vi "Data Parsing.vi"(8 "error in":errorcluster, 10 "Data Read":string, 11 "Modbus in":refnum<class "Modbus.lvclass">) -> (0 "error out":errorcluster, 1 "Graph Data":T1, 2 "Data Out":string[](array[string]), 3 "Modbus out":refnum<class "Modbus.lvclass">)   [LabVIEW 2021, in "Modbus.lvclass"]
uses:
  Modbus.lvclass
  controls/Data for Graph.ctl
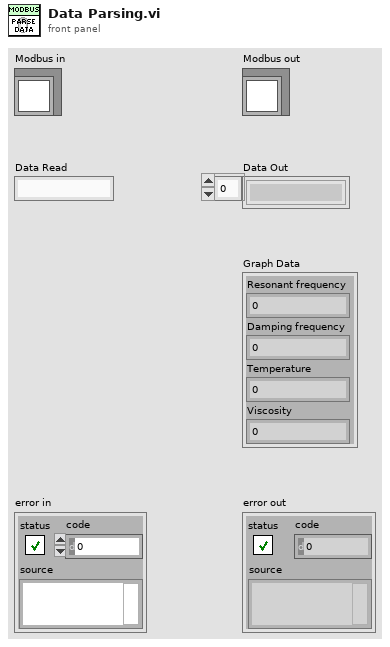
[diagram p1: front panel]
types:
  T1 = typedef "Data for Graph.ctl" = cluster{"Resonant frequency":dbl, "Damping frequency":dbl, "Temperature":dbl, "Viscosity":dbl}
  T2 = enum16{"big-endian, network order", "native, host order", "little-endian"}
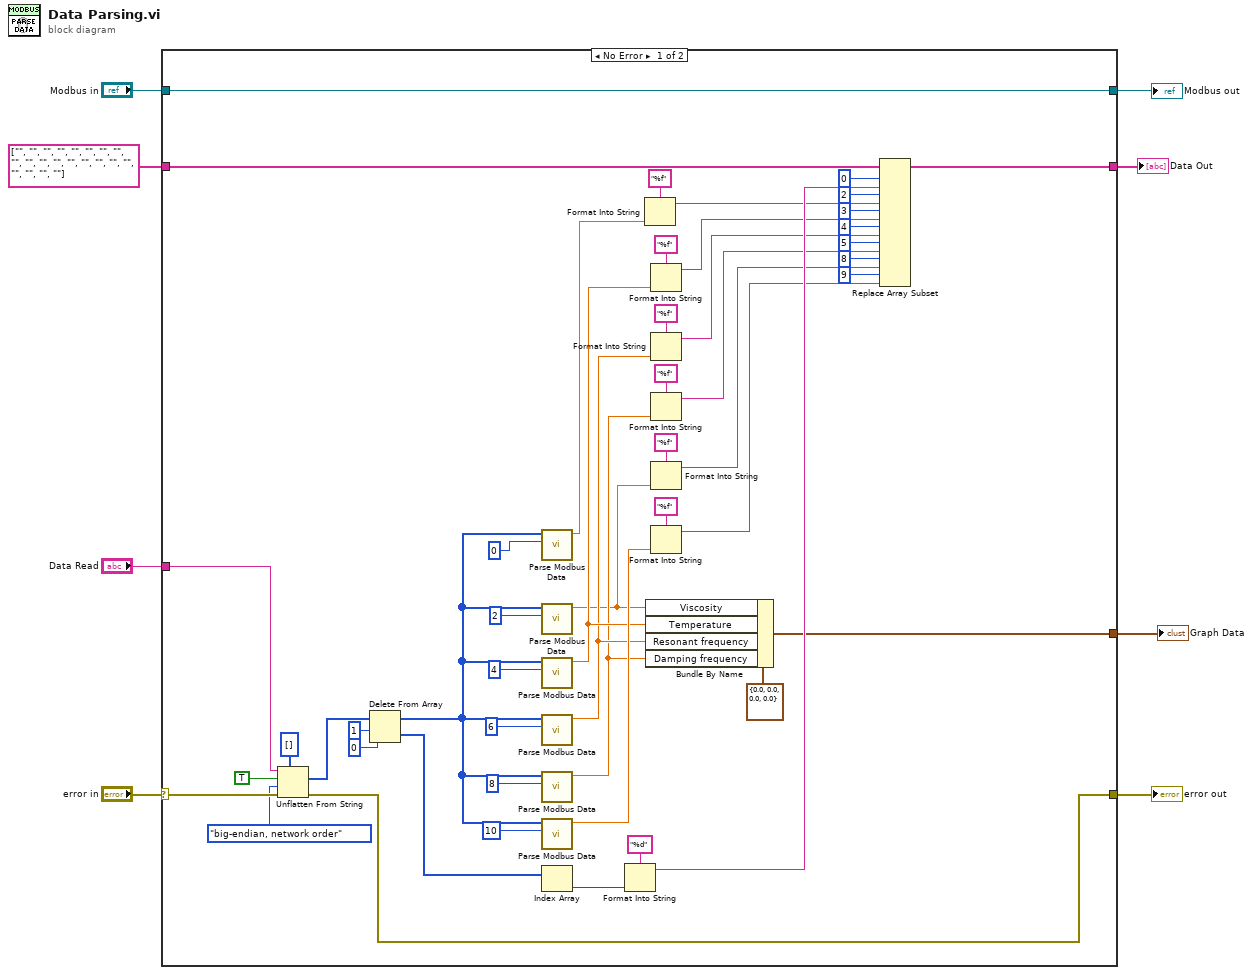
[diagram p0: block diagram]
diagram:
  n1 = case shown="No Error" "error in" {
    selector: "error in" -> [w53 w59]
    tunnel: [w38 w59] -> w7
    tunnel: "Modbus in" -> [w56 w60]
    tunnel: [w56 w60] -> w5
    tunnel: "Data Read" -> [w55 _]
    tunnel: [w39 _] -> w3
    tunnel: string[] ["", "", "", "", "", "", "", "", "", "", "", "", "", "", "", "", "", "", "", "", ""] -> [w37 _]
    tunnel: [w16 _] -> w1
    frame No Error {
      n2 = Unflatten From String(type=u16[] [] ("register values"), binary string=w55, data includes array or string size? (T)=TRUE, byte order (0:big-endian, network order)=T2."big-endian, network order", error in (no error)=w53) -> (value=w50:u16[], error out=w38:errorcluster)  [unwired: 1 out]
      n3 = Delete From Array(array=w50, length=1, index=0) -> (deleted portion=w36:u16[], array with subset deleted=w42:u16[])
      n4 = call "Parse Modbus Data.vi"("Start Index"=0, "Register Data"=w42) -> ("Result"=w32:dbl)  [unwired: 9 in]
      n5 = call "Parse Modbus Data.vi"("Start Index"=2, "Register Data"=w42) -> ("Result"=w19:dbl)  [unwired: 9 in]
      n6 = call "Parse Modbus Data.vi"("Start Index"=4, "Register Data"=w42) -> ("Result"=w25:dbl)  [unwired: 9 in]
      n7 = call "Parse Modbus Data.vi"("Start Index"=6, "Register Data"=w42) -> ("Result"=w24:dbl)  [unwired: 9 in]
      n8 = call "Parse Modbus Data.vi"("Start Index"=8, "Register Data"=w42) -> ("Result"=w23:dbl)  [unwired: 9 in]
      n9 = call "Parse Modbus Data.vi"("Start Index"=10, "Register Data"=w42) -> ("Result"=w57:dbl)  [unwired: 9 in]
      n10 = Index Array(array=w36) -> (element=w35:u16)  [unwired: 1 in]
      n11 = Format Into String(format string="%d", w35) -> (resulting string=w58:string)  [unwired: 2 in, 1 out]
      n12 = Format Into String(format string="%f", w32) -> (resulting string=w31:string)  [unwired: 2 in, 1 out]
      n13 = Bundle By Name(cluster=T1 {"Resonant frequency"=0.0, "Damping frequency"=0.0, "Temperature"=0.0, "Viscosity"=0.0} ("Graph Data"), "Viscosity"=w19, "Temperature"=w25, "Resonant frequency"=w24, "Damping frequency"=w23) -> (w39:T1)
      n14 = Format Into String(format string="%f", w25) -> (resulting string=w29:string)  [unwired: 2 in, 1 out]
      n15 = Format Into String(format string="%f", w24) -> (resulting string=w27:string)  [unwired: 2 in, 1 out]
      n16 = Format Into String(format string="%f", w23) -> (resulting string=w22:string)  [unwired: 2 in, 1 out]
      n17 = Format Into String(format string="%f", w19) -> (resulting string=w18:string)  [unwired: 2 in, 1 out]
      n18 = Format Into String(format string="%f", w57) -> (resulting string=w17:string)  [unwired: 2 in, 1 out]
      n19 = Replace Array Subset(array=w37, new element #1=w58, index #1=0 ("index"), new element #2=w31, index #2=2 ("index"), new element #3=w29, index #3=3 ("index"), new element #4=w27, index #4=4 ("index"), new element #5=w22, index #5=5 ("index"), new element #6=w18, index #6=8 ("index"), new element #7=w17, index #7=9 ("index")) -> (w16:string[])
    }
    frame Error {
    }
  }
  "error out" <- w7
  "Modbus out" <- w5
  "Data Out" <- w1
  "Graph Data" <- w3
